vi "Cached Read I32.vi"(8 "error in (no error)":errorcluster, 10 "CVT_I32 in":refnum<class "CVT_I32.lvclass">, 11 "Current Value Table in":refnum<class "Current Value Table.lvclass">) -> (0 "error out":errorcluster, 2 "value":i32, 3 "Current Value Table out":refnum<class "Current Value Table.lvclass">)   [LabVIEW 2024, in "Current Value Table.lvlib" / "Current Value Table.lvclass"]
uses:
  Current Value Table.lvclass
  Current Value Table.lvclass/Current Value Table.ctl
  CVT_I32/CVT_I32.lvclass
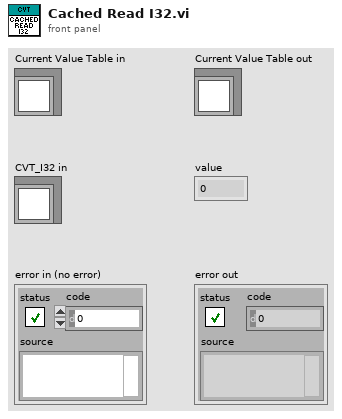
[diagram p1: front panel]
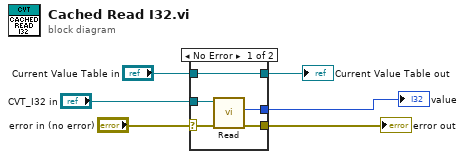
[diagram p0: block diagram]
diagram:
  n1 = case shown="No Error" "error in (no error)" {
    selector: "error in (no error)" -> [w8 w13]
    tunnel: [w7 w13] -> w5
    tunnel: [w11 w12] -> w3
    tunnel: "Current Value Table in" -> [w11 w12]
    tunnel: "CVT_I32 in" -> [w10 _]
    tunnel: [w9 _] -> w1
    frame No Error {
      n2 = call "Read.vi"("error in (no error)"=w8, "CVT_I32 in"=w10) -> ("error out"=w7:errorcluster, "value"=w9:i32)  [unwired: 7 in, 1 out]
    }
    frame Error {
    }
  }
  "error out" <- w5
  "Current Value Table out" <- w3
  "value" <- w1
